vi "libtiff2_open_w.vi"(8 "error in (no error)":errorcluster, 11 "Input path":path) -> (0 "error out":errorcluster, 3 "handle":i32)   [LabVIEW 2012]
doc: "Open a file for writing"
uses:
  C:/Program Files (x86)/GnuWin32/bin/libtiff3.dll
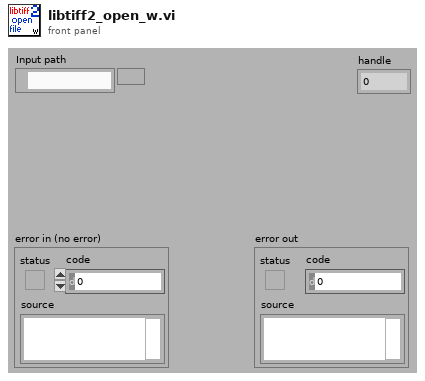
[diagram p1: front panel]
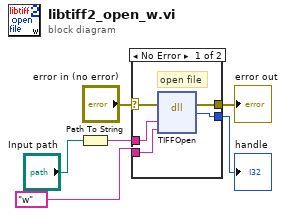
[diagram p0: block diagram]
diagram:
  n1 = Path To String(path="Input path") -> (string=w6:string)
  n2 = case shown="No Error" "error in (no error)" {
    selector: "error in (no error)" -> [w7 w12]
    tunnel: w6 -> [w11 _]
    tunnel: [w10 _] -> w4
    tunnel: "w" ("Mode") -> [w9 _]
    tunnel: [w8 w12] -> w2
    frame No Error {
      # "open file"
      n3 = dll-call lib="C:/Program Files (x86)/GnuWin32/bin/libtiff3.dll" fn="TIFFOpen"(error in=w7, "Filename"=w11, "Mode"=w9) -> (error out=w8:errorcluster, "return type"=w10:i32)  [unwired: 3 in, 2 out]
    }
    frame Error {
    }
  }
  "handle" <- w4
  "error out" <- w2
